vi "LcWebView_PolarPlot_Example.vi"() -> ()   [LabVIEW 2018, in "LcWebView.lvclass"]
doc: "Inject javascript arguments"
uses:
  LcWebView.lvclass
  D:/GitProjects/Public/GitHub/LcWebView/data/Microsoft.Web.WebView2.WinForms.dll
  data/Microsoft.Web.WebView2.WinForms.dll
  plots/ctrls/PlotType.ctl
  plots/ctrls/GenericPlotOption.ctl
  plots/ctrls/LegendPosition.ctl
panel:
  out "BrowserProcessId":u32
  out "Status Message":string
  in  "stop":bool
  in  "Web":refnum<k24>(container)
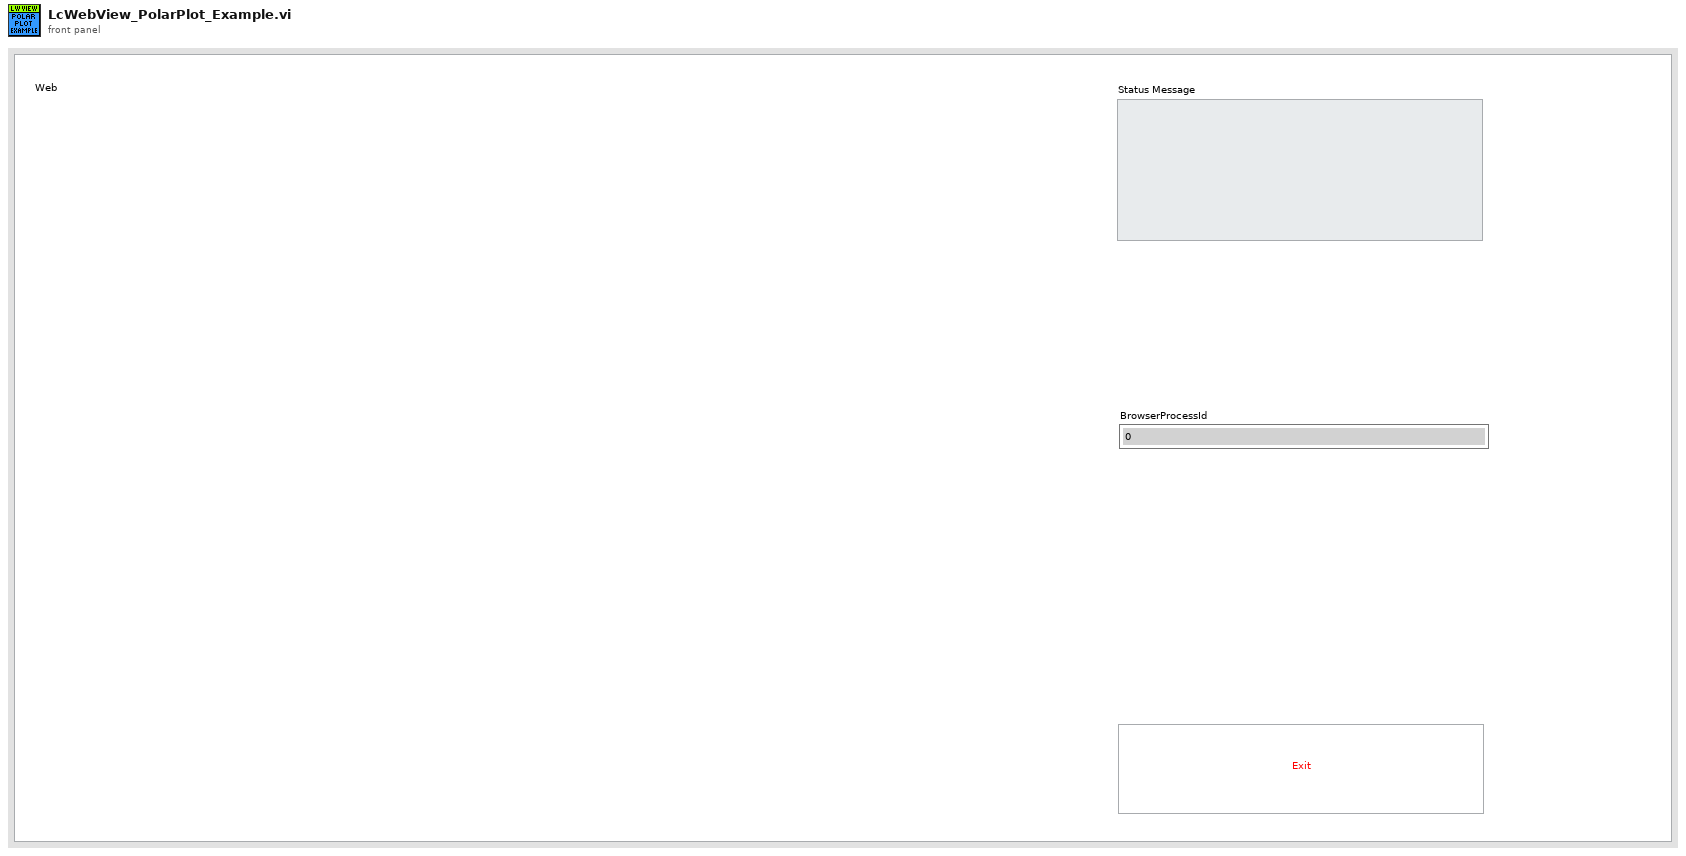
[diagram p1: front panel]
types:
  T1 = typedef "LcWebView.lvclass/GenericPlotOption.ctl" = cluster{"GraphTitle":string, "LegendDisplay":bool, "LegendPosition":T2}
  T2 = typedef "LcWebView.lvclass/LegendPosition.ctl" = enum16{"top", "right", "left", "bottom"}
  T3 = typedef "LcWebView.lvclass/PlotType.ctl" = enum16{"bar", "line", "pie", "doughnut", "scatter", "radar", "bubble", "polarArea"}
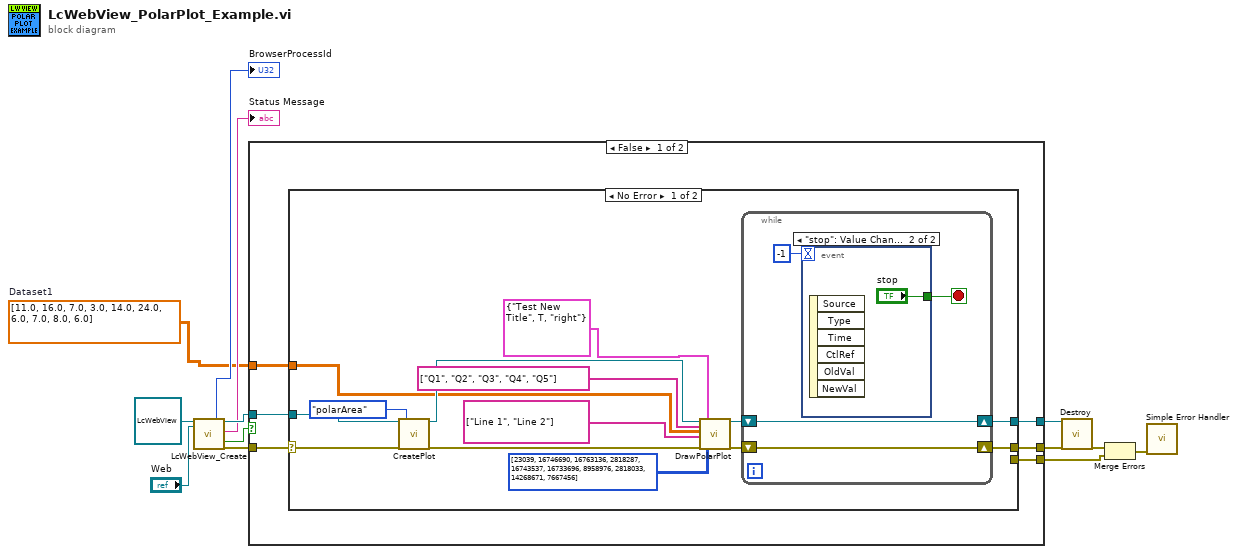
[diagram p0: block diagram]
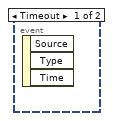
[diagram p2: hidden frame]
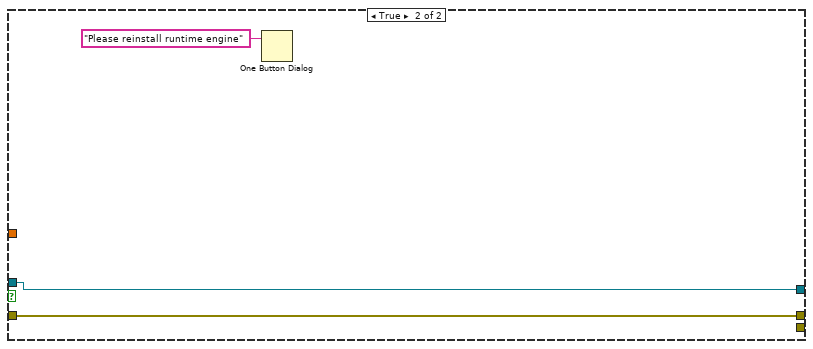
[diagram p4: hidden frame]
diagram:
  w1 = dbl[][] [[11.0, 16.0, 7.0, 3.0, 14.0], [24.0, 6.0, 7.0, 8.0, 6.0]]  # Dataset1
  n1 = call "LcWebView_Create.vi"("reference in"=refnum<class "LcWebView.lvclass"> refnum, "Webview container"="Web") -> ("BrowserProcessId"=→"BrowserProcessId":u32, "reference out"=w11:refnum<class "LcWebView.lvclass">, "Status Message"=→"Status Message":string, "Reinstall Runtime"=w4:bool, "Error Out"=w10:errorcluster)  [unwired: 10 in, 3 out]
  n2 = case shown="False" w4 {
    tunnel: w11 -> [w19 w43]
    tunnel: w10 -> [w18 w42]
    tunnel: [w17 w43] -> w9
    tunnel: [w15 w42] -> w8
    tunnel: [w16 _] -> w5
    tunnel: w1 -> [w14 _]
    frame False {
      n3 = case shown="No Error" w18 {
        selector: w18 -> [w31 w39]
        tunnel: w19 -> [w32 w40]
        tunnel: [w30 w40] -> w17
        tunnel: [w33 _] -> w15
        tunnel: [_ w39] -> w16
        tunnel: w14 -> [w28 _]
        frame No Error {
          n4 = call-dynamic "CreatePlot.vi"("reference in"=w32, "Error In"=w31, "PlotType"=PlotType."polarArea") -> ("reference out"=w29:refnum<class "LcWebView.lvclass">, "Error Out"=w25:errorcluster)  [unwired: 15 in]
          n5 = call-dynamic "DrawPolarPlot.vi"("reference in"=w29, "XLabels"=string[] ["Q1", "Q2", "Q3", "Q4", "Q5"], "Polar.Dataset"=w28, "LinePlot.DatasetLabels"=string[] ["Line 1", "Line 2"] ("DatasetLabels"), "Error In"=w25, "GenericPlotOptions"=T1 {"GraphTitle"="Test New Title", "LegendDisplay"=TRUE, "LegendPosition"=enum."right"}, "BarPlot.PlotColours"=u32[][] [[23039, 16746690, 16763136, 2818287, 16743537], [16733696, 8958976, 2818033, 14268671, 7667456]] ("PlotColours")) -> ("reference out"=w27:refnum<class "LcWebView.lvclass">, "Error Out"=w26:errorcluster)  [unwired: 11 in]
          n6 = while {
            shift-right: [w37] -> w30
            shift-left: w27 -> [w37]
            shift-right: [w36] -> w33
            shift-left: w26 -> [w36]
            stop <- w34 stop-if-true
            n7 = event shown="[1] \"stop\": Value Change" {
              selector: _ -> [_ _]
              dyn-events: _ -> [_ _]
              timeout: -1 -> [_ _]
              tunnel: [_ "stop"] -> w34
              event Timeout {
                n8 = event-data() -> ()  [unwired: 1 in, 3 out]
              }
              event "stop": Value Change {
                n9 = event-data() -> ()  [unwired: 1 in, 6 out]
              }
            }
          }
        }
        frame Error {
        }
      }
    }
    frame True {
      n10 = One Button Dialog(message="Please reinstall runtime engine") -> ()  [unwired: 1 in, 1 out]
    }
  }
  n11 = call-dynamic "Destroy.vi"("reference in"=w9, "Error In"=w8) -> ("Error Out"=w7:errorcluster)  [unwired: 16 in, 1 out]
  n12 = Merge Errors(w7, w5) -> (w2:errorcluster)
  n13 = call <vilib>:"Simple Error Handler.vi"("error in (no error)"=w2) -> ()  [unwired: 4 in, 5 out]
